vi "getLN2Level.vi"(8 "error in (no error)":errorcluster, 11 "Instrument.Cryostat in":refnum<class "Instrument.Cryostat.lvclass">) -> (0 "error out":errorcluster, 2 "LN2 Level (%)":dbl, 3 "Instrument.Cryostat out":refnum<class "Instrument.Cryostat.lvclass">)   [LabVIEW 2019, in "Instrument.Cryostat.lvclass"]
uses:
  Instrument.Cryostat.lvclass
  Typedefs/Cryostat.commands--enum.ctl
  Instrument/Instrument.lvclass
  14efb9d9-c5ba-40fa-a903-9fa1aad67bbf.vi
  C:/Users/patrick/Documents/GitHub/Instrument-Framework/lvsrc/Framework/Instrument/Instrument.lvclass
  C:/Program Files (x86)/National Instruments/LabVIEW 2019/vi.lib/JKI/JKI SMO/SMO/SMO.lvclass
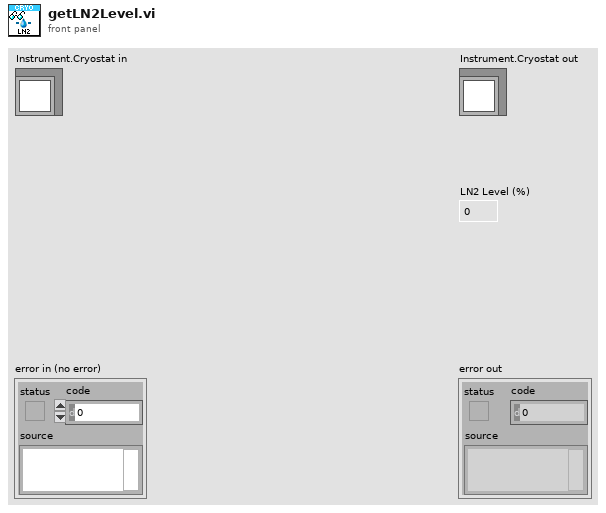
[diagram p1: front panel]
types:
  T1 = typedef "Instrument.Cryostat.lvclass/Cryostat.commands--enum.ctl" = enum16{"getLN2Level", "getLHeLevel", "getMagnet", "getMagnetVector", "setMagnet", "setMagnetVector", "getAngle", "setAngle", "getTemperature", "setTemperature", "getHeater", "setHeater", "getChamber", "setChamber", "getPressure"}
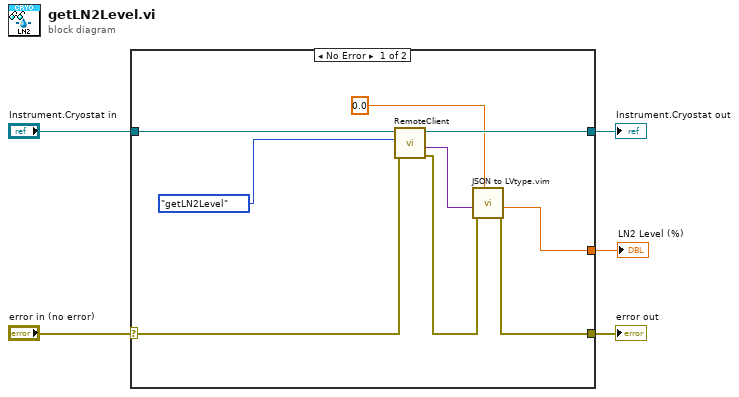
[diagram p0: block diagram]
diagram:
  n1 = case shown="No Error" "error in (no error)" {
    selector: "error in (no error)" -> [w11 w15]
    tunnel: [w14 w16] -> w3
    tunnel: "Instrument.Cryostat in" -> [w12 w16]
    tunnel: [w6 _] -> w2
    tunnel: [w8 w15] -> w1
    frame No Error {
      n2 = call "RemoteClient.vi"("error in (no error)"=w11, "Command in"=Cryostat.commands--enum."getLN2Level" ("commands"), "Instrument in"=w12) -> ("error out"=w9:errorcluster, "Data out"=w7:variant, "Instrument out"=w14:refnum<class "Instrument.Cryostat.lvclass">)  [unwired: 5 in, 1 out]
      n3 = call "JSON to LVtype.vim"("type"=0.0, "error in (no error)"=w9, "JSON Data in"=w7) -> ("error out"=w8:errorcluster, "Data out"=w6:dbl)  [unwired: 7 in]
    }
    frame Error {
    }
  }
  "error out" <- w1
  "Instrument.Cryostat out" <- w3
  "LN2 Level (%)" <- w2
